vi "GOOP_SetWindowsRegistry.vi"(8 "error in (no error)":errorcluster, 10 "ExeFile":path, 11 "IconFile":path) -> (0 "error out":errorcluster)   [LabVIEW 2014]
uses:
  <vilib>/registry/registry.llb/Registry RtKey.ctl
  <vilib>/registry/registry.llb/Read Registry Value Simple STR.vi
  <vilib>/registry/registry.llb/Write Registry Value Simple STR.vi
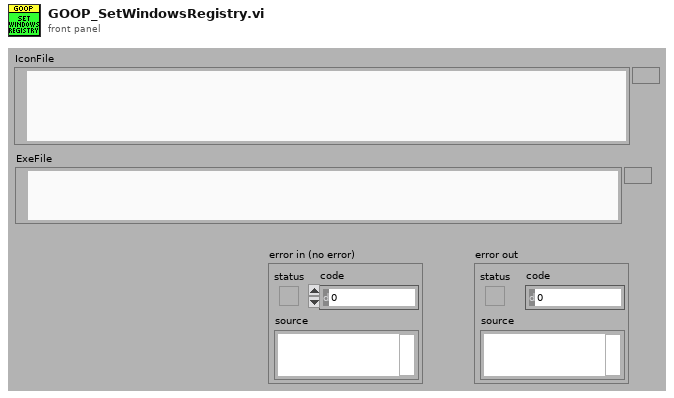
[diagram p1: front panel]
types:
  T1 = typedef "Registry RtKey.ctl" = enum32{"HKEY_CLASSES_ROOT", "HKEY_CURRENT_USER", "HKEY_LOCAL_MACHINE", "HKEY_USERS", "HKEY_PERFORMANCE_DATA", "HKEY_CURRENT_CONFIG", "HKEY_DYN_DATA"}
  T2 = typedef "Registry refnum.ctl" = refnum<k1>
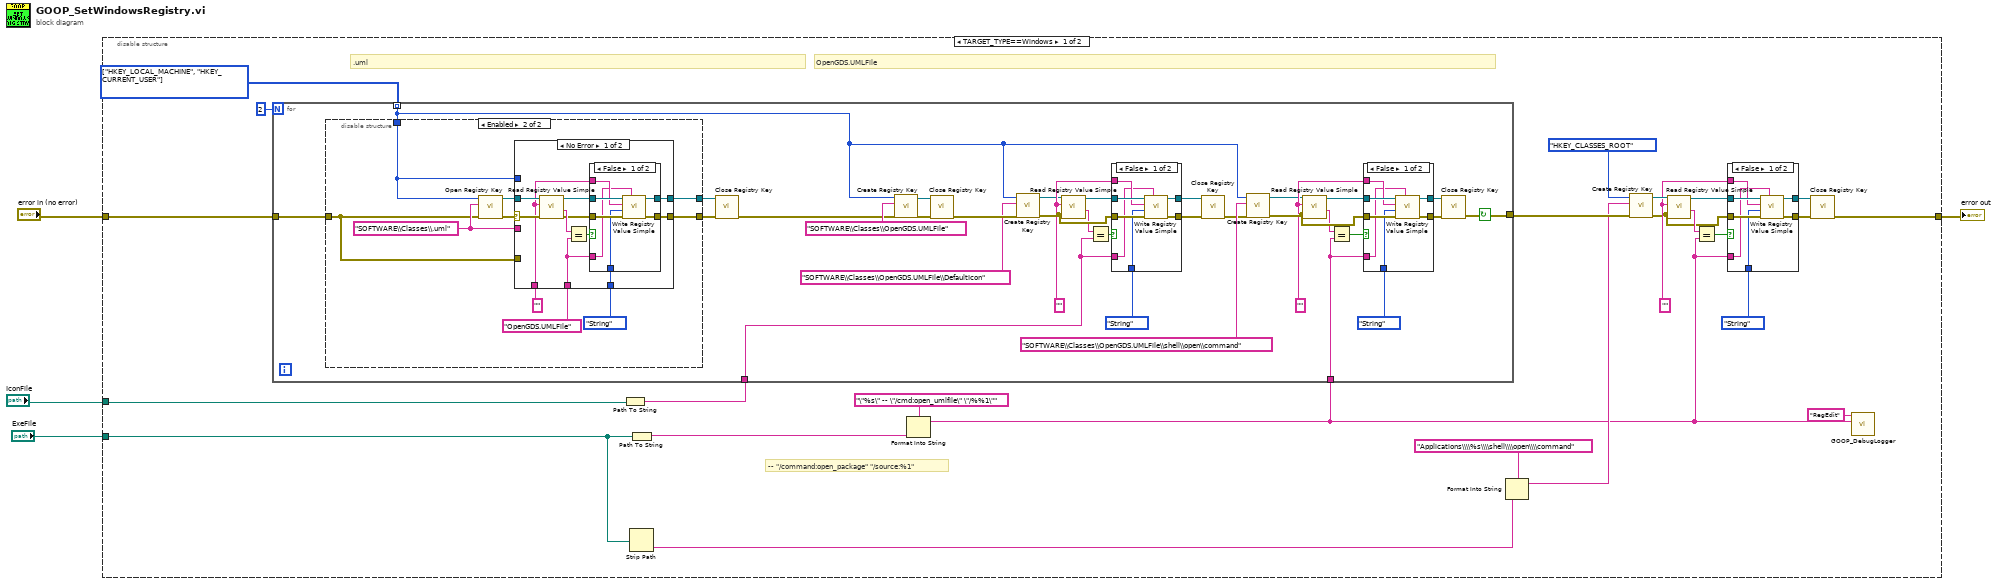
[diagram p0: block diagram]
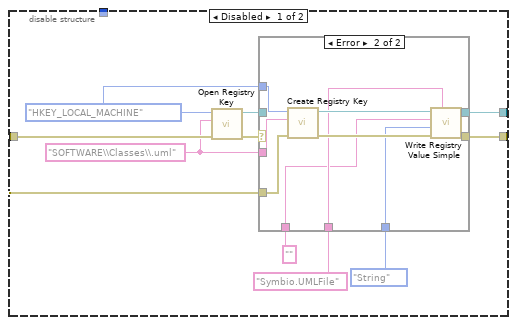
[diagram p4: hidden frame]
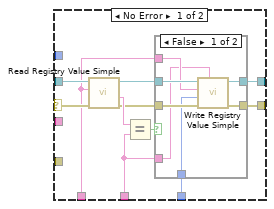
[diagram p5: hidden frame]
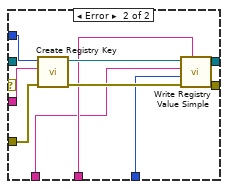
[diagram p8: hidden frame]
diagram:
  n1 = disable-structure shown="TARGET_TYPE==Windows" {
    disable-tunnel: [w16 _] -> w4
    disable-tunnel: "ExeFile" -> [w6 _]
    disable-tunnel: "IconFile" -> [w15 _]
    disable-tunnel: "error in (no error)" -> [w14 _]
    frame condition #0 (active) {
      w11 = T1[] [enum."HKEY_LOCAL_MACHINE", enum."HKEY_CURRENT_USER"] items=["HKEY_CLASSES_ROOT", "HKEY_CURRENT_USER", "HKEY_LOCAL_MACHINE", "HKEY_USERS", "HKEY_PERFORMANCE_DATA", "HKEY_CURRENT_CONFIG", "HKEY_DYN_DATA"]
      w22 = "" ("value")
      # "-- \"/command:open_package\" \"/source:%1\""
      # "OpenGDS.UMLFile"
      # ".uml"
      n2 = Path To String(path=w15) -> (string=w27:string)
      n3 = Path To String(path=w6) -> (string=w28:string)
      n4 = Strip Path(path=w6) -> (name=w5:string)  [unwired: 1 out]
      n5 = Format Into String(format string="\"%s\" -- \"/cmd:open_umlfile\" \"/%%1\"", w28) -> (resulting string=w7:string)  [unwired: 2 in, 1 out]
      n6 = for {
        N: 2 -> [_]
        tunnel: w27 -> [w44]
        tunnel: [w30] -> w17
        tunnel: w7 -> [w33]
        tunnel: w14 -> [w32]
        tunnel: w11 -> [w31] mode=indexing
        stop <- w30 continue-if-true
        w57 = "" ("value")
        w43 = "" ("value")
        n7 = disable-structure shown="Enabled" {
          disable-tunnel: w32 -> [w89 w122]
          disable-tunnel: [w83 w125] -> w34
          disable-tunnel: [w82 w124] -> w35
          disable-tunnel: w31 -> [_ w121]
          frame Disabled {
            w87 = "SOFTWARE\\Classes\\.uml" ("subkey")
            w88 = Registry_RtKey."HKEY_LOCAL_MACHINE" ("root key (HKEY_LOCAL_MACHINE)")
            n8 = call <vilib>:"Open Registry Key.vi"("error in (no error)"=w89, "subkey"=w87, "root key (HKEY_LOCAL_MACHINE)"=w88) -> ("error out"=w90:errorcluster, "refnum out"=w86:T2)  [unwired: 7 in]
            n9 = case shown="Error" w90 {
              selector: w90 -> [w101 _]
              tunnel: w89 -> [_ w120]
              tunnel: w88 -> [_ w119]
              tunnel: w87 -> [_ w118]
              tunnel: w86 -> [w100 _]
              tunnel: "Symbio.UMLFile" ("y") -> [w95 w113]
              tunnel: "" ("value") -> [w94 w112]
              tunnel: [w93 w114] -> w83
              tunnel: [w92 w115] -> w82
              tunnel: enum16{"String", "Binary", "DWORD"}."String" ("simple data type") -> [w91 w111]
              frame No Error {
                n10 = call-poly <vilib>:"Read Registry Value Simple.vi"("error in (no error)"=w101, "value"=w94, "refnum"=w100) -> ("error out"=w97:errorcluster, "String/Binary data"=w99:string, "refnum out"=w96:T2)  [unwired: 3 in, 1 out]
                n11 = Equal?(x=w99, y=w95) -> (x = y?=w98:bool)
                n12 = case shown="False" w98 {
                  tunnel: w97 -> [w108 w110]
                  tunnel: w96 -> [w107 w109]
                  tunnel: w94 -> [w104 _]
                  tunnel: w95 -> [w103 _]
                  tunnel: [w105 w110] -> w93
                  tunnel: [w106 w109] -> w92
                  tunnel: w91 -> [w102 _]
                  frame False {
                    n13 = call-poly <vilib>:"Write Registry Value Simple.vi"("String/Binary data"=w103, "error in (no error)"=w108, "simple data type"=w102, "value"=w104, "refnum"=w107) -> ("error out"=w105:errorcluster, "refnum out"=w106:T2)  [unwired: 3 in]
                  }
                  frame True {
                  }
                }
              }
              frame Error {
                n14 = call <vilib>:"Create Registry Key.vi"("error in (no error)"=w120, "subkey"=w118, "root key (HKEY_LOCAL_MACHINE)"=w119) -> ("error out"=w116:errorcluster, "refnum out"=w117:T2)  [unwired: 6 in, 1 out]
                n15 = call-poly <vilib>:"Write Registry Value Simple.vi"("String/Binary data"=w113, "error in (no error)"=w116, "simple data type"=w111, "value"=w112, "refnum"=w117) -> ("error out"=w114:errorcluster, "refnum out"=w115:T2)  [unwired: 3 in]
              }
            }
          }
          frame Enabled {
            w129 = "SOFTWARE\\Classes\\.uml" ("subkey")
            n16 = call <vilib>:"Open Registry Key.vi"("error in (no error)"=w122, "subkey"=w129, "root key (HKEY_LOCAL_MACHINE)"=w121) -> ("error out"=w130:errorcluster, "refnum out"=w128:T2)  [unwired: 7 in]
            n17 = case shown="No Error" w130 {
              selector: w130 -> [w141 _]
              tunnel: w122 -> [_ w160]
              tunnel: w121 -> [_ w159]
              tunnel: w129 -> [_ w158]
              tunnel: w128 -> [w140 _]
              tunnel: "OpenGDS.UMLFile" ("y") -> [w135 w153]
              tunnel: "" ("value") -> [w134 w152]
              tunnel: [w133 w154] -> w125
              tunnel: [w132 w155] -> w124
              tunnel: enum16{"String", "Binary", "DWORD"}."String" ("simple data type") -> [w131 w151]
              frame No Error {
                n18 = call-poly <vilib>:"Read Registry Value Simple.vi"("error in (no error)"=w141, "value"=w134, "refnum"=w140) -> ("error out"=w137:errorcluster, "String/Binary data"=w139:string, "refnum out"=w136:T2)  [unwired: 3 in, 1 out]
                n19 = Equal?(x=w139, y=w135) -> (x = y?=w138:bool)
                n20 = case shown="False" w138 {
                  tunnel: w137 -> [w148 w150]
                  tunnel: w136 -> [w147 w149]
                  tunnel: w134 -> [w144 _]
                  tunnel: w135 -> [w143 _]
                  tunnel: [w145 w150] -> w133
                  tunnel: [w146 w149] -> w132
                  tunnel: w131 -> [w142 _]
                  frame False {
                    n21 = call-poly <vilib>:"Write Registry Value Simple.vi"("String/Binary data"=w143, "error in (no error)"=w148, "simple data type"=w142, "value"=w144, "refnum"=w147) -> ("error out"=w145:errorcluster, "refnum out"=w146:T2)  [unwired: 3 in]
                  }
                  frame True {
                  }
                }
              }
              frame Error {
                n22 = call <vilib>:"Create Registry Key.vi"("error in (no error)"=w160, "subkey"=w158, "root key (HKEY_LOCAL_MACHINE)"=w159) -> ("error out"=w156:errorcluster, "refnum out"=w157:T2)  [unwired: 6 in, 1 out]
                n23 = call-poly <vilib>:"Write Registry Value Simple.vi"("String/Binary data"=w153, "error in (no error)"=w156, "simple data type"=w151, "value"=w152, "refnum"=w157) -> ("error out"=w154:errorcluster, "refnum out"=w155:T2)  [unwired: 3 in]
              }
            }
          }
        }
        n24 = call <vilib>:"Close Registry Key.vi"("error in (no error)"=w34, "refnum"=w35) -> ("error out"=w37:errorcluster)  [unwired: 5 in]
        n25 = call <vilib>:"Create Registry Key.vi"("error in (no error)"=w37, "subkey"="SOFTWARE\\Classes\\OpenGDS.UMLFile", "root key (HKEY_LOCAL_MACHINE)"=w31) -> ("error out"=w48:errorcluster, "refnum out"=w49:T2)  [unwired: 6 in, 1 out]
        n26 = call <vilib>:"Close Registry Key.vi"("error in (no error)"=w48, "refnum"=w49) -> ("error out"=w50:errorcluster)  [unwired: 5 in]
        n27 = call <vilib>:"Create Registry Key.vi"("error in (no error)"=w50, "subkey"="SOFTWARE\\Classes\\OpenGDS.UMLFile\\DefaultIcon", "root key (HKEY_LOCAL_MACHINE)"=w31) -> ("error out"=w61:errorcluster, "refnum out"=w42:T2)  [unwired: 6 in, 1 out]
        n28 = call-poly <vilib>:"Read Registry Value Simple.vi"("error in (no error)"=w61, "value"=w43, "refnum"=w42) -> ("String/Binary data"=w41:string, "refnum out"=w39:T2)  [unwired: 3 in, 2 out]
        n29 = Equal?(x=w41, y=w44) -> (x = y?=w40:bool)
        n30 = case shown="False" w40 {
          tunnel: w61 -> [w78 w80]
          tunnel: w39 -> [w77 w79]
          tunnel: w43 -> [w74 _]
          tunnel: w44 -> [w73 _]
          tunnel: [w75 w80] -> w46
          tunnel: [w76 w79] -> w47
          tunnel: enum16{"String", "Binary", "DWORD"}."String" ("simple data type") -> [w72 _]
          frame False {
            n31 = call-poly <vilib>:"Write Registry Value Simple.vi"("String/Binary data"=w73, "error in (no error)"=w78, "simple data type"=w72, "value"=w74, "refnum"=w77) -> ("error out"=w75:errorcluster, "refnum out"=w76:T2)  [unwired: 3 in]
          }
          frame True {
          }
        }
        n32 = call <vilib>:"Close Registry Key.vi"("error in (no error)"=w46, "refnum"=w47) -> ("error out"=w51:errorcluster)  [unwired: 5 in]
        n33 = call <vilib>:"Create Registry Key.vi"("error in (no error)"=w51, "subkey"="SOFTWARE\\Classes\\OpenGDS.UMLFile\\shell\\open\\command", "root key (HKEY_LOCAL_MACHINE)"=w31) -> ("error out"=w62:errorcluster, "refnum out"=w54:T2)  [unwired: 6 in, 1 out]
        n34 = call-poly <vilib>:"Read Registry Value Simple.vi"("error in (no error)"=w62, "value"=w57, "refnum"=w54) -> ("String/Binary data"=w53:string, "refnum out"=w56:T2)  [unwired: 3 in, 2 out]
        n35 = Equal?(x=w53, y=w33) -> (x = y?=w55:bool)
        n36 = case shown="False" w55 {
          tunnel: w62 -> [w69 w71]
          tunnel: w56 -> [w68 w70]
          tunnel: w57 -> [w65 _]
          tunnel: w33 -> [w64 _]
          tunnel: [w66 w71] -> w59
          tunnel: [w67 w70] -> w60
          tunnel: enum16{"String", "Binary", "DWORD"}."String" ("simple data type") -> [w63 _]
          frame False {
            n37 = call-poly <vilib>:"Write Registry Value Simple.vi"("String/Binary data"=w64, "error in (no error)"=w69, "simple data type"=w63, "value"=w65, "refnum"=w68) -> ("error out"=w66:errorcluster, "refnum out"=w67:T2)  [unwired: 3 in]
          }
          frame True {
          }
        }
        n38 = call <vilib>:"Close Registry Key.vi"("error in (no error)"=w59, "refnum"=w60) -> ("error out"=w30:errorcluster)  [unwired: 5 in]
      }
      n39 = Format Into String(format string="Applications\\\\%s\\\\shell\\\\open\\\\command" ("value"), w5) -> (resulting string=w9:string)  [unwired: 2 in, 1 out]
      n40 = call <vilib>:"Create Registry Key.vi"("error in (no error)"=w17, "subkey"=w9, "root key (HKEY_LOCAL_MACHINE)"=Registry_RtKey."HKEY_CLASSES_ROOT") -> ("error out"=w18:errorcluster, "refnum out"=w25:T2)  [unwired: 6 in, 1 out]
      n41 = call-poly <vilib>:"Read Registry Value Simple.vi"("error in (no error)"=w18, "value"=w22, "refnum"=w25) -> ("String/Binary data"=w26:string, "refnum out"=w23:T2)  [unwired: 3 in, 2 out]
      n42 = Equal?(x=w26, y=w7) -> (x = y?=w24:bool)
      n43 = case shown="False" w24 {
        tunnel: w18 -> [w167 w169]
        tunnel: w23 -> [w166 w168]
        tunnel: w22 -> [w163 _]
        tunnel: w7 -> [w162 _]
        tunnel: [w164 w169] -> w20
        tunnel: [w165 w168] -> w19
        tunnel: enum16{"String", "Binary", "DWORD"}."String" ("simple data type") -> [w161 _]
        frame False {
          n44 = call-poly <vilib>:"Write Registry Value Simple.vi"("String/Binary data"=w162, "error in (no error)"=w167, "simple data type"=w161, "value"=w163, "refnum"=w166) -> ("error out"=w164:errorcluster, "refnum out"=w165:T2)  [unwired: 3 in]
        }
        frame True {
        }
      }
      n45 = call <vilib>:"Close Registry Key.vi"("error in (no error)"=w20, "refnum"=w19) -> ("error out"=w16:errorcluster)  [unwired: 5 in]
      n46 = call <resource>:"GOOP_DebugLogger.vi"("Data"=w7, "State"="RegEdit") -> ()  [unwired: 8 in, 2 out]
    }
    frame condition #1 {
    }
  }
  "error out" <- w4
